vi "Set DAC (Volts).vi"(7 "Channel Select":T1, 8 "error in (no error)":errorcluster, 10 "DAC Output (V)":dbl, 11 "DAC8552 in":refnum<class "LINX-DAC8552.lvclass">) -> (0 "error out":errorcluster, 3 "DAC8552 out":refnum<class "LINX-DAC8552.lvclass">)   [LabVIEW 2020, in "LINX-DAC8552.lvclass"]
doc: "Enables the DAC8552 and sets the DAC voltage according to the formula: Vout = Vref * D/65536"
uses:
  LINX-DAC8552.lvclass
  Channel Select.ctl
  LINX-DAC8552.lvclass/LINX-DAC8552.ctl
  Read VRef.vi
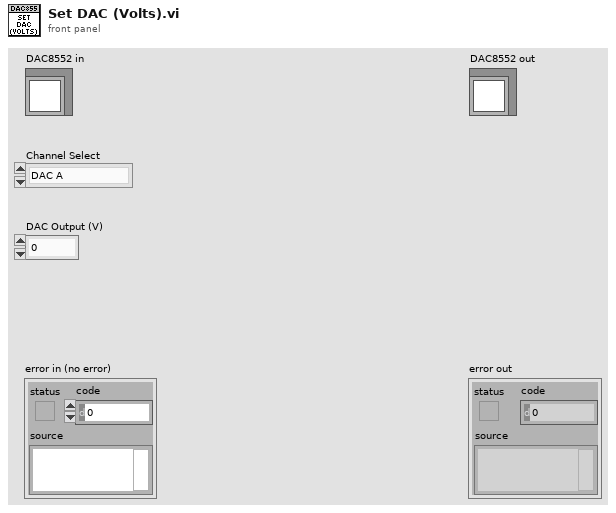
[diagram p1: front panel]
types:
  T1 = typedef "LINX-DAC8552.lvclass/Channel Select.ctl" = enum8{"DAC A", "DAC B", "Both"}
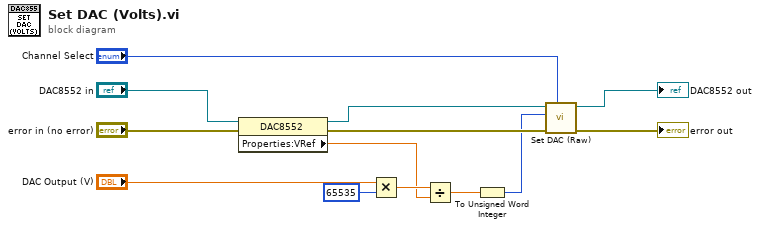
[diagram p0: block diagram]
diagram:
  n1 = property class="DAC8552"(reference="DAC8552 in", error in="error in (no error)") -> (reference out=w8:refnum<class "LINX-DAC8552.lvclass">, error out=w10:errorcluster, "Properties:VRef"=w3:dbl)
  n2 = Multiply(x="DAC Output (V)", y=u16 65535) -> (x*y=w4:dbl)
  n3 = Divide(x=w4, y=w3) -> (x/y=w2:dbl)
  n4 = To Unsigned Word Integer(number=w2) -> (unsigned 16bit integer=w1:u16)
  n5 = call "Set DAC (Raw).vi"("Channel Select"="Channel Select", "error in (no error)"=w10, "DAC Value (Raw)"=w1, "DAC8552 in"=w8) -> ("error out"=→"error out":errorcluster, "DAC8552 out"=→"DAC8552 out":refnum<class "LINX-DAC8552.lvclass">)  [unwired: 6 in]
